vi "host_chunk (PXI).vi"() -> ()   [LabVIEW 2020]
doc: "This example demonstrates how to continuously acquire buffered voltage measurements using a DAQmx device.\n\nFor instructions on how to connect your signals to the DAQ device, refer to your device documentation."
uses:
  <vilib>/DAQmx/read.llb/DAQmx Read (Analog Wfm 1Chan NSamp).vi
  <vilib>/DAQmx/create/channels.llb/DAQmx Create Channel (AI-Voltage-Basic).vi
  <vilib>/DAQmx/configure/timing.llb/DAQmx Timing (Sample Clock).vi
  <vilib>/Utility/error.llb/Error Cluster From Error Code.vi
  <vilib>/rvi/errors/niLvFpgaAdjustHostInterfaceError.vi
  <vilib>/FPGAPlugInAG/Dynamic/niLvFpga_Run_Dynamic.vi
  <vilib>/RVI Host/nirviSupport.llb/nirviErrorClusterFromErrorCode.vi
  <vilib>/DAQmx/miscellaneous.llb/DAQmx Fill In Error Info.vi
  <vilib>/FPGAPlugInAG/Dynamic/niLvFpga_Close_Dynamic.vi
  <vilib>/rvi/interface/nirviOpenFPGA/nirviOpenFPGA.xnode
  <vilib>/rvi/interface/nirviReadWriteControl/nirviReadWriteControl.xnode
  <vilib>/rvi/interface/nirviMethod/nirviMethod.xnode
  <vilib>/rvi/interface/nirviCloseFPGA/nirviCloseFPGA.xnode
  <resource>/objmgr/daqmx.rc
  <vilib>/rvi/interface/Simulation/niFpgaSimulationCallBeginRW.vi
  <vilib>/rvi/errors/niLvFpgaMergeErrorWithErrorCode.vi
  NiFpgaLv.dll
  <vilib>/FPGAPlugInAG/Dynamic/niLvFpga_WriteFifo_Dynamic.vi
  <vilib>/FPGAPlugInAG/Dynamic/niLvFpga_ReadFifo_Dynamic.vi
  <vilib>/rvi/interface/nirviMethod/StockFPGA_InlinedMethodWaitForSingleIRQ.vi
  <vilib>/FPGAPlugInAG/Dynamic/niLvFpga_WaitOnIrq_Dynamic.vi
  <vilib>/FPGAPlugInAG/Dynamic/niLvFpga_AcknowledgeIrq_Dynamic.vi
  FPGA Bitfiles/testDMA_7858_chunk_v1002.lvbitx
  <vilib>/FPGAPlugInAG/PXIe-7858R/niLvFpga_Open_PXIe-7858R.vi
  <vilib>/rvi/interface/common/dynamic/niFpgaDynamicAddResources.vi
panel:
  in  "DMA read per cycle (1)":i32=16
  out "dma read time uS":u32
  out "AvailSampPerChan":u32
  out "write DMA timeout count":i16
  out "uS elapsed":cluster{u32, u32}(graph)
  out "Timed Out":bool
  out "error out":errorcluster
  in  "Stop":bool
  out "Waveform Graph":dbl[][](graph)
  in  "Number of Samples":i32=100
  in  "Sample Rate":dbl=1000.0
  in  "Sample Clock Source":tag="OnboardClock"
  in  "Terminal Configuration":i32(ring)=-1 items=["default"=-1, "RSE"=10083, "NRSE"=10078, "Differential"=10106, "Pseudodifferential"=12529]
  in  "Max Voltage":dbl=5.0
  in  "Min Voltage":dbl=-5.0
  in  "Physical Channel":tag="PXI1Slot3/ai0"
  out "Actual Sample Rate":dbl=1000.0 format="%0.2f"
  # "Channel Settings"
  # "Acquired Data"
  # "Timing Settings"
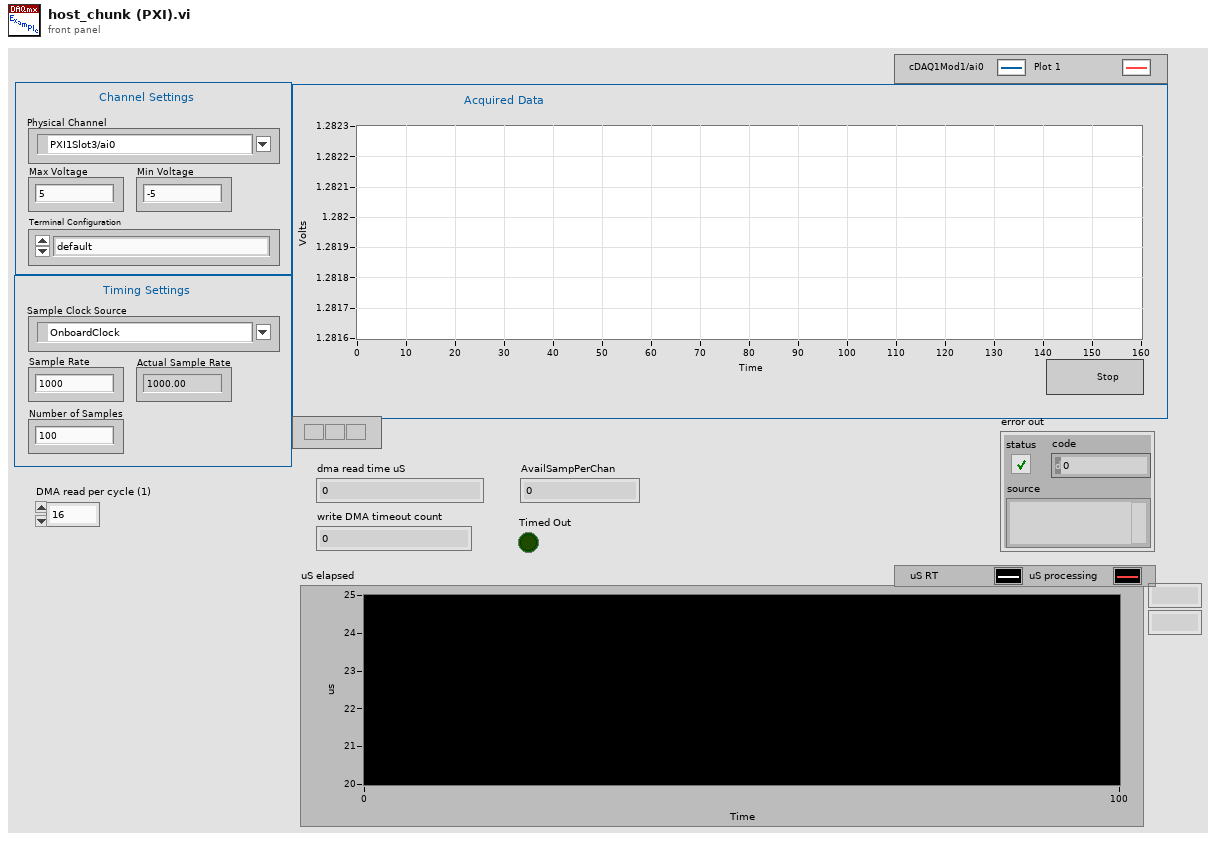
[diagram p1: front panel]
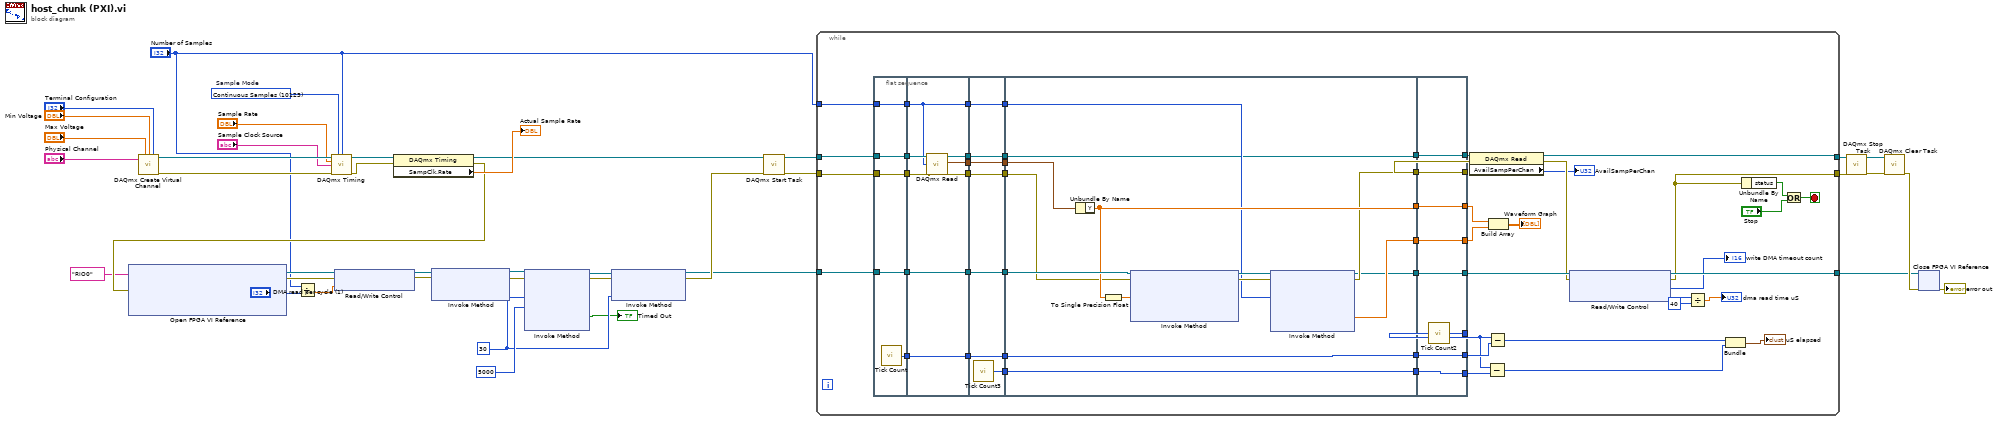
[diagram p0: block diagram]
diagram:
  w7 = u8 30 ("IRQ Number (0)")
  w38 = 10123 items=["Finite Samples"=10178, "Continuous Samples"=10123, "Hardware Timed Single Point"=12522]  # Sample Mode
  n1 = call-poly <vilib>:"DAQmx Create Virtual Channel.vi"("maximum value"="Max Voltage", "minimum value"="Min Voltage", "input terminal configuration"="Terminal Configuration", "physical channels"="Physical Channel") -> ("task out"=w36:refnum<k21>, "error out"=w37:errorcluster)  [unwired: 10 in]
  n2 = Divide(x="Number of Samples", y="DMA read per cycle (1)") -> (x/y=w2:dbl)
  n3 = call-poly <vilib>:"DAQmx Timing.vi"("task/channels in"=w36, "sample mode"=w38, "samples per channel"="Number of Samples", "rate"="Sample Rate", "source"="Sample Clock Source", "error in"=w37) -> ("task out"=w40:refnum<k21>, "error out"=w39:errorcluster)  [unwired: 8 in]
  n4 = property class="DAQmx Timing"(reference=w40, error in=w39) -> (reference out=w19:refnum<k21>, error out=w20:errorcluster, "SampClk.Rate"=→"Actual Sample Rate":dbl)
  n5 = xnode "Open FPGA VI Reference"("error in"=w20, "resource name"=tag "RIO0") -> ("FPGA VI Reference Out"=w17:refnum<k20>, "error out"=w18:errorcluster)
  n6 = xnode "Read/Write Control"("FPGA VI Reference In"=w17, "error in"=w18, "number of samples"=w2) -> ("FPGA VI Reference Out"=w14:refnum<k20>, "error out"=w13:errorcluster)
  n7 = xnode "Invoke Method"("FPGA VI Reference In"=w14, "error in"=w13) -> ("FPGA VI Reference Out"=w12:refnum<k20>, "error out"=w11:errorcluster)  [unwired: 1 in]
  n8 = xnode "Invoke Method"("FPGA VI Reference In"=w12, "error in"=w11, "IRQ Number(s)"=w7, "Timeout (ms)"=5000) -> ("FPGA VI Reference Out"=w10:refnum<k20>, "error out"=w9:errorcluster, "Timed Out"=→"Timed Out":bool)  [unwired: 1 out]
  n9 = xnode "Invoke Method"("FPGA VI Reference In"=w10, "error in"=w9, "IRQ Number(s)"=w7) -> ("FPGA VI Reference Out"=w4:refnum<k20>, "error out"=w5:errorcluster)
  n10 = call <vilib>:"DAQmx Start Task.vi"("task/channels in"=w19, "error in"=w5) -> ("task out"=w35:refnum<k21>, "error out"=w34:errorcluster)  [unwired: 12 in]
  n11 = while {
    tunnel: w35 -> [w93]
    tunnel: w34 -> [w88]
    tunnel: [w70] -> w26
    tunnel: [w73] -> w25
    tunnel: "Number of Samples" -> [w58]
    tunnel: w4 -> [w87]
    tunnel: [w74] -> w3
    stop <- w89 stop-if-true
    n12 = flat-sequence {
      tunnel: w93 -> [w98]
      tunnel: [w98] -> w63
      tunnel: [w97] -> w62
      tunnel: w88 -> [w97]
      tunnel: [w96] -> w61
      tunnel: w87 -> [w96]
      tunnel: [w95] -> w60
      tunnel: [w94] -> w59
      tunnel: w58 -> [w94]
      tunnel: w63 -> [w104]
      tunnel: [w104] -> w57
      tunnel: w62 -> [w103]
      tunnel: [w103] -> w55
      tunnel: w61 -> [w102]
      tunnel: [w102] -> w53
      tunnel: w60 -> [w101]
      tunnel: [w101] -> w51
      tunnel: [w100] -> w49
      tunnel: w59 -> [w99]
      tunnel: [w99] -> w47
      tunnel: w57 -> [w111]
      tunnel: [w111] -> w56
      tunnel: w55 -> [w110]
      tunnel: [w110] -> w54
      tunnel: w53 -> [w109]
      tunnel: [w109] -> w52
      tunnel: w51 -> [w108]
      tunnel: [w108] -> w50
      tunnel: w49 -> [w107]
      tunnel: [w107] -> w48
      tunnel: w47 -> [w106]
      tunnel: [w106] -> w46
      tunnel: [w105] -> w42
      tunnel: w56 -> [w113]
      tunnel: w54 -> [w114]
      tunnel: w52 -> [w125]
      tunnel: [w113] -> w82
      tunnel: [w119] -> w81
      tunnel: [w121] -> w80
      tunnel: [w120] -> w79
      tunnel: [w118] -> w78
      tunnel: [w117] -> w76
      tunnel: w50 -> [w117]
      tunnel: w48 -> [w116]
      tunnel: w46 -> [w115]
      tunnel: [w112] -> w43
      tunnel: w42 -> [w112]
      tunnel: [w129] -> w83
      tunnel: [w130] -> w86
      tunnel: [w131] -> w85
      tunnel: [w132] -> w69
      tunnel: [w133] -> w92
      tunnel: w82 -> [w133]
      tunnel: w81 -> [w132]
      tunnel: w80 -> [w131]
      tunnel: w79 -> [w130]
      tunnel: w78 -> [w129]
      tunnel: [w128] -> w45
      tunnel: [w127] -> w77
      tunnel: w76 -> [w127]
      tunnel: [w126] -> w44
      tunnel: w43 -> [w126]
      frame #0 {
        n13 = call "Tick Count"() -> ("Tick Count(uSec)"=w95:u32)
      }
      frame #1 {
        n14 = call-poly <vilib>:"DAQmx Read.vi"("task/channels in"=w104, "number of samples per channel"=w99, "error in"=w103) -> ("data"=w100:waveform(dbl))  [unwired: 10 in, 2 out]
      }
      frame #2 {
        n15 = call "Tick Count3"() -> ("Tick Count(uSec)"=w105:u32)
      }
      frame #3 {
        n16 = Unbundle By Name(w116) -> ("Y"=w120:dbl[])
        n17 = To Single Precision Float(number=w120) -> (single precision float=w124:sgl[])
        n18 = xnode "Invoke Method"("FPGA VI Reference In"=w125, "error in"=w114, "Data"=w124) -> ("FPGA VI Reference Out"=w123:refnum<k20>, "error out"=w122:errorcluster)  [unwired: 1 in, 1 out]
        n19 = xnode "Invoke Method"("FPGA VI Reference In"=w123, "error in"=w122, "Number of Elements"=w115) -> ("FPGA VI Reference Out"=w118:refnum<k20>, "error out"=w119:errorcluster, "Data"=w121:sgl[])  [unwired: 1 in, 1 out]
      }
      frame #4 {
        n20 = call "Tick Count2"() -> ("Tick Count(uSec)"=w128:u32)
      }
    }
    n21 = property class="DAQmx Read"(reference=w92, error in=w69) -> (reference out=w70:refnum<k21>, error out=w68:errorcluster, "AvailSampPerChan"=→"AvailSampPerChan":u32)
    n22 = Subtract(x=w45, y=w44) -> (x-y=w41:u32)
    n23 = Subtract(x=w45, y=w77) -> (x-y=w75:u32)
    n24 = Build Array(w86, w85) -> (→"Waveform Graph":dbl[][])
    n25 = xnode "Read/Write Control"("FPGA VI Reference In"=w83, "error in"=w68) -> ("FPGA VI Reference Out"=w74:refnum<k20>, "error out"=w73:errorcluster, "write DMA timeout count"=→"write DMA timeout count":i16, "dma read time ticks"=w66:u32)
    n26 = Divide(x=w66, y=u32 40) -> (x/y=→"dma read time uS":dbl)
    n27 = Bundle(w75, w41) -> (→"uS elapsed":cluster{u32, u32})  [unwired: 1 in]
    n28 = Unbundle By Name(w73) -> ("status"=w90:bool)
    n29 = Or(x=w90, y="Stop") -> (x .or. y?=w89:bool)
  }
  n30 = call <vilib>:"DAQmx Stop Task.vi"("task/channels in"=w26, "error in"=w25) -> ("task out"=w23:refnum<k21>, "error out"=w24:errorcluster)  [unwired: 12 in]
  n31 = call <vilib>:"DAQmx Clear Task.vi"("task in"=w23, "error in"=w24) -> ("error out"=w22:errorcluster)  [unwired: 13 in]
  n32 = xnode "Close FPGA VI Reference"("FPGA VI Reference In"=w3, "error in"=w22) -> ("error out"=→"error out":errorcluster)
